vi "String_Display.vi"(10 "error in (no error)":errorcluster, 11 "USB Interface Name":refnum<visa-resource-name>="COM3") -> (1 "error out":errorcluster, 2 "String Out":string, 3 "VISA resource name out":refnum<visa-resource-name>="COM1")   [LabVIEW 2012]
panel:
  out "actual bytes read":u32
  out "Bytes to read":u32
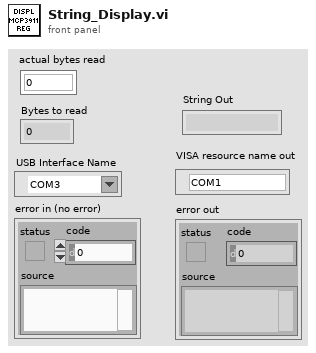
[diagram p1: front panel]
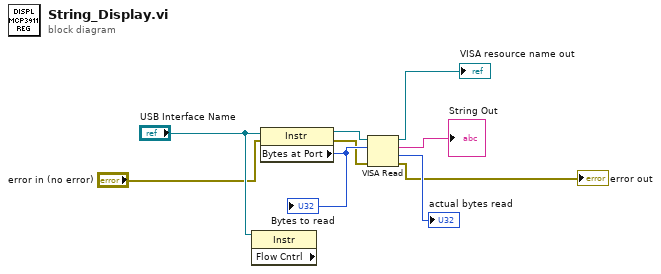
[diagram p0: block diagram]
diagram:
  n1 = property class="Instr" props=["Flow Cntrl"](reference="USB Interface Name") -> ()  [unwired: 1 in, 3 out]
  n2 = property class="Instr"(reference="USB Interface Name", error in="error in (no error)") -> (reference out=w9:refnum<visa-resource-name>, error out=w6:errorcluster, "Bytes at Port"=w7:u32)
  "Bytes to read" <- w7
  n3 = VISA Read(VISA resource name=w9, byte count=w7, error in (no error)=w6) -> (VISA resource name out=→"VISA resource name out":refnum<visa-resource-name>, read buffer=→"String Out":string, return count=→"actual bytes read":u32, error out=→"error out":errorcluster)
